vi "Create.vi"(8 "error in (no error)":errorcluster, 9 "Player2Name":string, 10 "Player1Name":string, 11 "InitialBoard":refnum<class "Board.lvclass">) -> (0 "error out":errorcluster, 3 "GameRecorder out":refnum<class "GameRecorder.lvclass">)   [LabVIEW 2015, in "TronviewGame.lvlib" / "GameRecorder.lvclass"]
uses:
  GameRecorder.lvclass
  Board/Board.lvclass
  GameRecorder.lvclass/GameRecorder.ctl
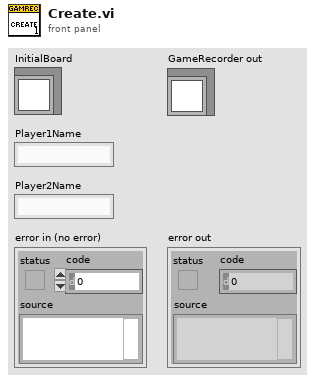
[diagram p1: front panel]
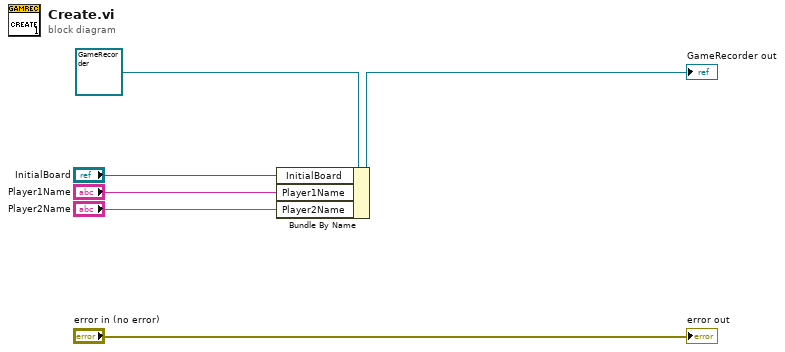
[diagram p0: block diagram]
diagram:
  n1 = Bundle By Name(cluster=refnum<class "GameRecorder.lvclass"> refnum ("GameRecorder in"), "InitialBoard"="InitialBoard", "Player1Name"="Player1Name", "Player2Name"="Player2Name") -> (→"GameRecorder out":refnum<class "GameRecorder.lvclass">)
  "error out" <- "error in (no error)"
